vi "data table to subtable.vi"(11 "full data table":T2) -> (3 "subtable":T1)   [LabVIEW 2013, in "Tag Bus Web Interface configuration.lvclass"]
uses:
  Tag Bus Web Interface configuration.lvclass
  <vilib>/NI/Tag Bus/table/data table.ctl
  subtable.ctl
  <vilib>/NI/Tag Bus/table/data table.lvlib
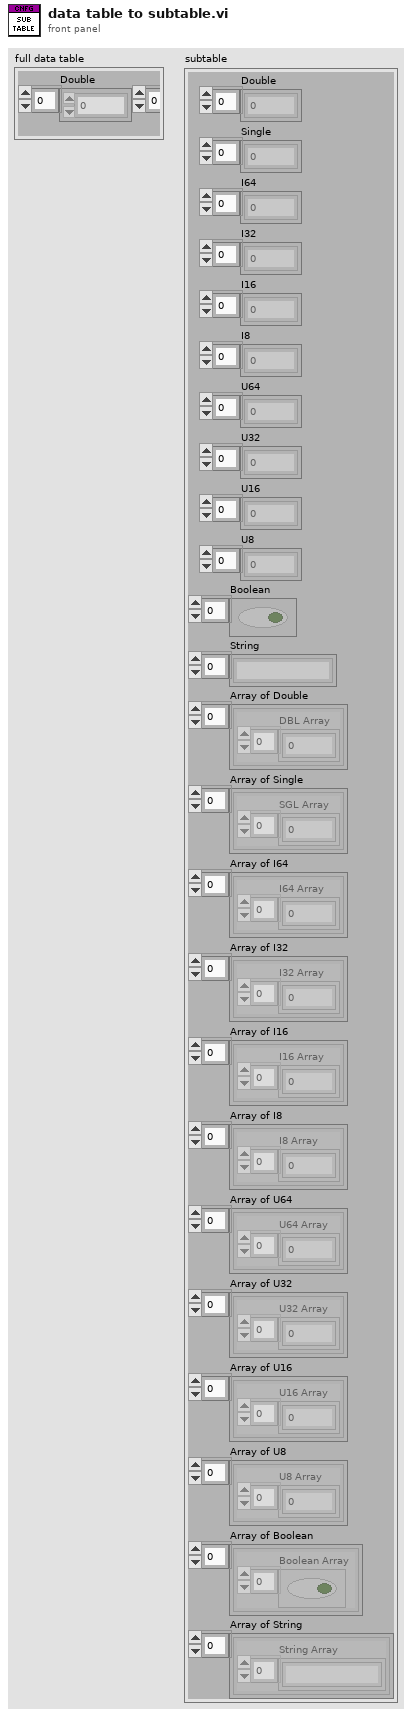
[diagram p1: front panel]
types:
  T1 = typedef "Tag Bus Web Interface configuration.lvclass/subtable.ctl" = cluster{"Double":dbl[], "Single":sgl[], "I64":i64[], "I32":i32[], "I16":i16[], "I8":i8[], "U64":u64[], "U32":u32[], "U16":u16[], "U8":u8[], "Boolean":bool[], "String":string[], "Array of Double":cluster{"DBL Array":dbl[]}[], "Array of Single":cluster{"SGL Array":sgl[]}[], "Array of I64":cluster{"I64 Array":i64[]}[], "Array of I32":cluster{"I32 Array":i32[]}[], "Array of I16":cluster{"I16 Array":i16[]}[], "Array of I8":cluster{"I8 Array":i8[]}[], "Array of U64":cluster{"U64 Array":u64[]}[], "Array of U32":cluster{"U32 Array":u32[]}[], "Array of U16":cluster{"U16 Array":u16[]}[], "Array of U8":cluster{"U8 Array":u8[]}[], "Array of Boolean":cluster{"Boolean Array":bool[]}[], "Array of String":cluster{"String Array":string[]}[]}
  T2 = typedef "tag bus.lvlib/data table.lvlib/data table.ctl" = cluster{"Double":dbl[], "Single":sgl[], "I64":i64[], "I32":i32[], "I16":i16[], "I8":i8[], "U64":u64[], "U32":u32[], "U16":u16[], "U8":u8[], "Boolean":bool[], "String":string[], "Array of Double":cluster{"DBL Array":dbl[]}[], "Array of Single":cluster{"SGL Array":sgl[]}[], "Array of I64":cluster{"I64 Array":i64[]}[], "Array of I32":cluster{"I32 Array":i32[]}[], "Array of I16":cluster{"I16 Array":i16[]}[], "Array of I8":cluster{"I8 Array":i8[]}[], "Array of U64":cluster{"U64 Array":u64[]}[], "Array of U32":cluster{"U32 Array":u32[]}[], "Array of U16":cluster{"U16 Array":u16[]}[], "Array of U8":cluster{"U8 Array":u8[]}[], "Array of Boolean":cluster{"Boolean Array":bool[]}[], "Array of String":cluster{"String Array":string[]}[]}
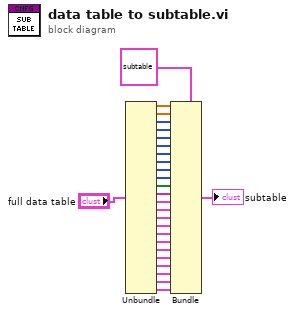
[diagram p0: block diagram]
diagram:
  n1 = Unbundle("full data table") -> ("Double"=w24:dbl[], "Single"=w23:sgl[], "I64"=w22:i64[], "I32"=w21:i32[], "I16"=w20:i16[], "I8"=w19:i8[], "U64"=w18:u64[], "U32"=w17:u32[], "U16"=w16:u16[], "U8"=w15:u8[], "Boolean"=w14:bool[], "String"=w13:string[], "Array of Double"=w12:cluster{"DBL Array":dbl[]}[], "Array of Single"=w11:cluster{"SGL Array":sgl[]}[], "Array of I64"=w10:cluster{"I64 Array":i64[]}[], "Array of I32"=w9:cluster{"I32 Array":i32[]}[], "Array of I16"=w8:cluster{"I16 Array":i16[]}[], "Array of I8"=w7:cluster{"I8 Array":i8[]}[], "Array of U64"=w6:cluster{"U64 Array":u64[]}[], "Array of U32"=w5:cluster{"U32 Array":u32[]}[], "Array of U16"=w4:cluster{"U16 Array":u16[]}[], "Array of U8"=w1:cluster{"U8 Array":u8[]}[], "Array of Boolean"=w3:cluster{"Boolean Array":bool[]}[], "Array of String"=w2:cluster{"String Array":string[]}[])
  n2 = Bundle(cluster=T1 {"Double"=[], "Single"=[], "I64"=[], "I32"=[], "I16"=[], "I8"=[], "U64"=[], "U32"=[], "U16"=[], "U8"=[], "Boolean"=[], "String"=[], "Array of Double"=[], "Array of Single"=[], "Array of I64"=[], "Array of I32"=[], "Array of I16"=[], "Array of I8"=[], "Array of U64"=[], "Array of U32"=[], "Array of U16"=[], "Array of U8"=[], "Array of Boolean"=[], "Array of String"=[]} ("full data table"), "Double"=w24, "Single"=w23, "I64"=w22, "I32"=w21, "I16"=w20, "I8"=w19, "U64"=w18, "U32"=w17, "U16"=w16, "U8"=w15, "Boolean"=w14, "String"=w13, "Array of Double"=w12, "Array of Single"=w11, "Array of I64"=w10, "Array of I32"=w9, "Array of I16"=w8, "Array of I8"=w7, "Array of U64"=w6, "Array of U32"=w5, "Array of U16"=w4, "Array of U8"=w1, "Array of Boolean"=w3, "Array of String"=w2) -> (→"subtable":T1)
